vi "Threshold Thing.vi"() -> ()   [LabVIEW 2014]
panel:
  out "Triggered":bool
  in  "Threshold":dbl
  in  "Slide Control":dbl(slide) scale=0.0..10.0
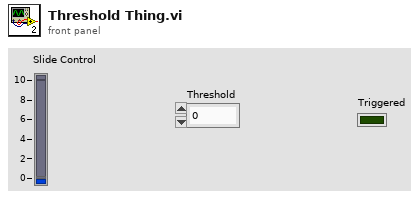
[diagram p1: front panel]
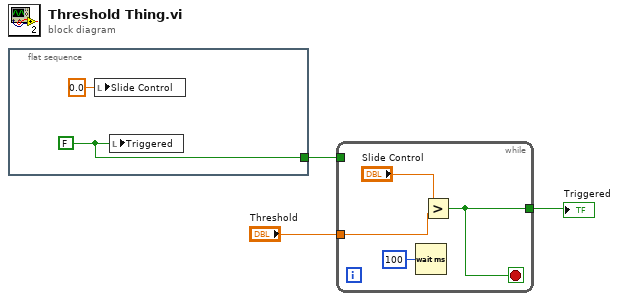
[diagram p0: block diagram]
diagram:
  n1 = flat-sequence {
    tunnel: [w4] -> w3
    frame #0 {
      w4 = FALSE
      n2 = local write "Slide Control"(0.0 ("Slide Control")) -> ()
      n3 = local write "Triggered"(w4) -> ()
    }
  }
  n4 = while {
    tunnel: w3 -> [_]
    tunnel: "Threshold" -> [w8]
    tunnel: [w7] -> w1
    stop <- w7 stop-if-true
    n5 = Wait (ms)(milliseconds to wait=u32 100) -> ()  [unwired: 1 out]
    n6 = Greater?(x="Slide Control", y=w8) -> (0:w7:bool)
  }
  "Triggered" <- w1
